vi "ZAlign_GroupAndMovetoBack.vi"(8 "error in (no error)":errorcluster, 10 "CtrlRefs":refnum<vi>[](array[refnum]) caption="Objects", 11 "Panel":refnum<vi>) -> (0 "error out":errorcluster)   [LabVIEW 2014, in "ZAlign.lvlib"]
doc: "ZAlign.lvlib:ZAlign_GroupAndMovetoBack.vi\n----------------------------------------------\nDecos group an move to Back\n\nInputs:\n---------------------\n- error in (no error) : Cluster; \n- Objects : 1DArrayOfRefnum; \n- Panel : Refnum; \n\nOutputs:\n---------------------\n- error out : Cluster; \n\n----------------------------------------------\n16/03/2015\nZühlke Engineering AG\nCH-8952 Schlieren\nwww.zuehlke.com"
uses:
  ZAlign.lvlib
panel:
  # "Connector Pane"
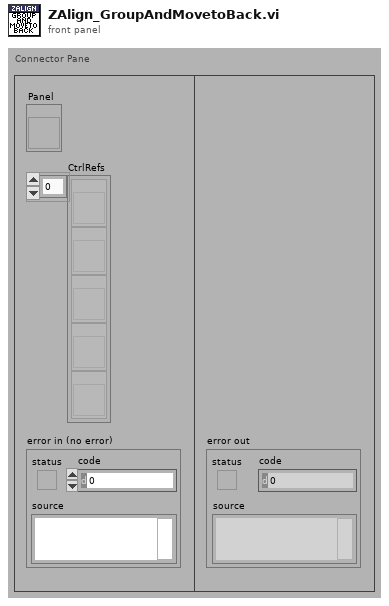
[diagram p1: front panel]
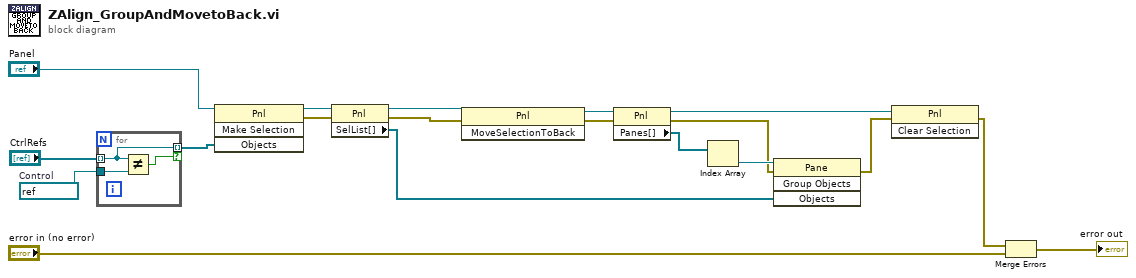
[diagram p0: block diagram]
diagram:
  w6 = refnum<vi> refnum  # Control
  n1 = for {
    tunnel: "CtrlRefs" -> [w21] mode=indexing
    tunnel: w6 -> [w22]
    tunnel: [w21] -> w4 mode=indexing if=w20
    n2 = Not Equal?(x=w21, y=w22) -> (x != y?=w20:bool)
  }
  n3 = invoke class="Pnl" method="Make Selection"(reference="Panel", "Objects"=w4) -> (reference out=w18:refnum<vi>, error out=w17:errorcluster)  [unwired: 2 in, 2 out]
  n4 = property class="Pnl"(reference=w18, error in=w17) -> (reference out=w16:refnum<vi>, error out=w15:errorcluster, "SelList[]"=w7:refnum<vi>[])
  n5 = invoke class="Pnl" method="MoveSelectionToBack"(reference=w16, error in=w15) -> (reference out=w13:refnum<vi>, error out=w14:errorcluster)  [unwired: 1 in, 1 out]
  n6 = property class="Pnl"(reference=w13, error in=w14) -> (reference out=w8:refnum<vi>, error out=w10:errorcluster, "Panes[]"=w12:refnum<vi>[])
  n7 = Index Array(array=w12) -> (element=w11:refnum<vi>)  [unwired: 1 in]
  n8 = invoke class="Pane" method="Group Objects"(reference=w11, error in=w10, "Objects"=w7) -> (error out=w9:errorcluster)  [unwired: 1 in, 3 out]
  n9 = invoke class="Pnl" method="Clear Selection"(reference=w8, error in=w9) -> (error out=w1:errorcluster)  [unwired: 1 in, 2 out]
  n10 = Merge Errors(w1, "error in (no error)") -> (→"error out":errorcluster)
